vi "Not_Used less than n days.vi"(8 "error in (no error)":errorcluster, 9 "days":dbl=180.0, 11 "element in":T1) -> (0 "error out":errorcluster, 3 "less than 180 days?":bool)   [LabVIEW 2012]
uses:
  typedef/User_Data_Cluster.ctl
  typedef/User Accounts.ctl
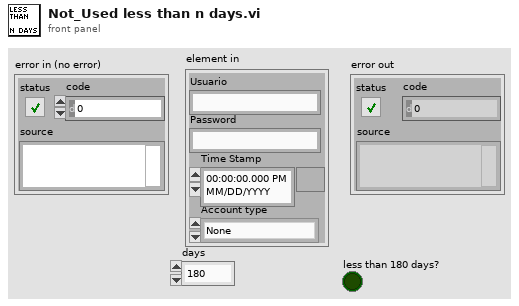
[diagram p1: front panel]
types:
  T1 = typedef "User_Data_Cluster.ctl" = cluster{"Usuario":string, "Password":string, "Account type":T2, "Time Stamp":timestamp}
  T2 = typedef "User Accounts.ctl" = enum16{"None", "User", "Admin"}
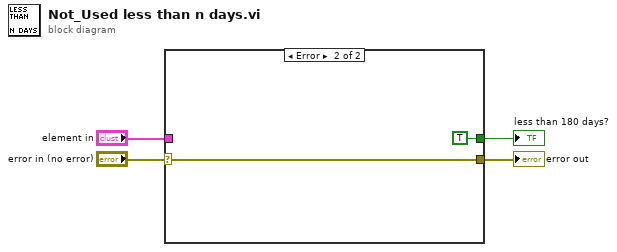
[diagram p0: block diagram]
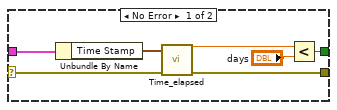
[diagram p2: hidden frame]
diagram:
  n1 = case shown="Error" "error in (no error)" {
    selector: "error in (no error)" -> [w5 w12]
    tunnel: "element in" -> [w8 _]
    tunnel: [w7 TRUE] -> w3
    tunnel: [w6 w12] -> w1
    frame No Error {
      n2 = Unbundle By Name(w8) -> ("Time Stamp"=w9:timestamp)
      n3 = call "Time_elapsed.vi"("error in (no error)"=w5, "From"=w9) -> ("error out"=w6:errorcluster, "Days"=w10:dbl)  [unwired: 6 in, 2 out]
      n4 = Less?(x=w10, y="days") -> (x < y?=w7:bool)
    }
    frame Error {
    }
  }
  "less than 180 days?" <- w3
  "error out" <- w1
